vi "自动填充.vi"(5 "填充方式":i32(ring)=1 items=["xlFillCopy"=1, "xlFillDays"=5, "xlFillDefault"=0, "xlFillFormats"=3, "xlFillMonths"=7, "xlFillSeries"=2, "xlFillValues"=4, "xlFillWeekdays"=6, "xlFillYears"=8, "xlGrowthTrend"=10, "xlLinearTrend"=9, "xlFlashFill"=11], 7 "工作表名称":string="Sheet1", 8 "错误输入（无错误）":errorcluster, 11 "单元格区域":T1={"起始列"="A", "起始行"=1, "大小"=[]} {"大小" min=1 max=1048576; "起始行" min=1 max=1048576}) -> (0 "错误输出":errorcluster)   [LabVIEW 2020, in "OperateExcel.lvlib"]
uses:
  OperateExcel.lvlib
  Globals.vi
  <vilib>/Utility/error.llb/Error Cluster From Error Code.vi
  <vilib>/ErrorRing/Error Ring.xnode
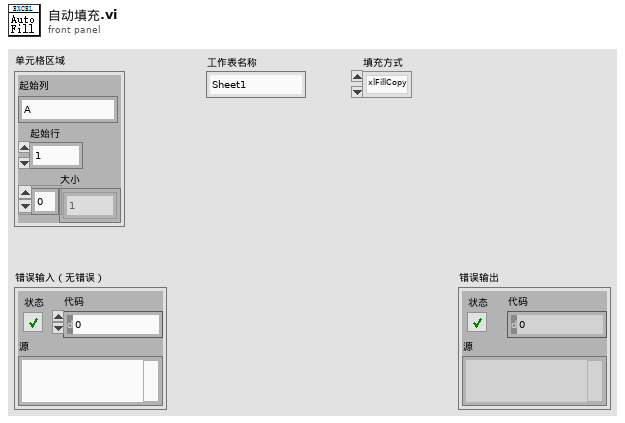
[diagram p1: front panel]
types:
  T1 = typedef "OperateExcel.lvlib/单元格区域.ctl" = cluster{"起始列":string, "起始行":u32, "大小":u32[]}
  T2 = typedef "OperateExcel.lvlib/引用簇.ctl" = cluster{"Excel._Application":refnum<k7>, "Workbooks":refnum<k7>, "Open":refnum<k7>, "Worksheets":refnum<k7>, "sheetList":refnum<k7>[]}
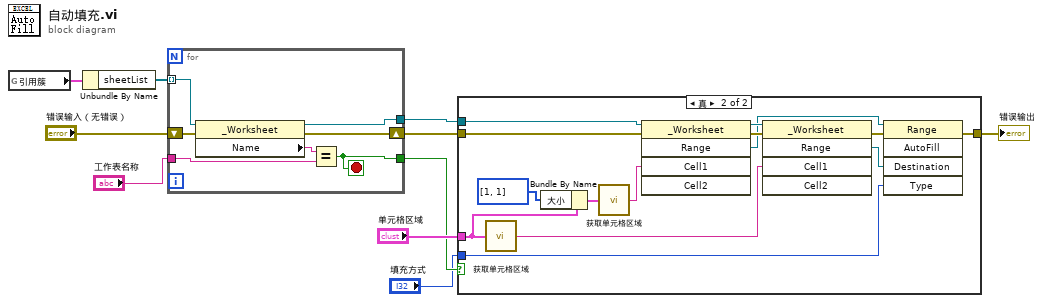
[diagram p0: block diagram]
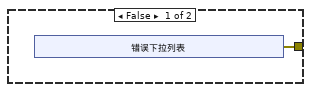
[diagram p2: hidden frame]
diagram:
  n1 = global read "Globals.vi" "引用簇"() -> (w3:T2)
  n2 = Unbundle By Name(w3) -> ("sheetList"=w10:refnum<k7>[])
  n3 = for {
    tunnel: w10 -> [w17] mode=indexing
    tunnel: "工作表名称" -> [w15]
    tunnel: [w14] -> w9
    shift-right: [w12] -> w7
    shift-left: "错误输入（无错误）" -> [w13]
    tunnel: [w11] -> w2
    stop <- w11 stop-if-true
    n4 = property class="_Worksheet"(reference=w17, error in=w13) -> (reference out=w14:refnum<k7>, error out=w12:errorcluster, "Name"=w16:string)
    n5 = Equal?(x=w16, y=w15) -> (x = y?=w11:bool)
  }
  n6 = case shown="真" w2 {
    tunnel: w9 -> [_ w32]
    tunnel: w7 -> [_ w26]
    tunnel: [w18 w35] -> w6
    tunnel: "单元格区域" -> [_ w30]
    tunnel: "填充方式" -> [_ w33]
    frame False {
      n7 = xnode "错误下拉列表"() -> ("错误输出"=w18:errorcluster)
    }
    frame True {
      n8 = call "获取单元格区域.vi"("单元格区域"=w30) -> ("单元格区域"=w34:string)
      n9 = Bundle By Name(cluster=w30, "大小"=u32[] [1, 1]) -> (w29:T1)
      n10 = call "获取单元格区域.vi"("单元格区域"=w29) -> ("单元格区域"=w27:string)
      n11 = invoke class="_Worksheet" method="Range"(reference=w32, error in=w26, "Cell1"=w27) -> (reference out=w31:refnum<k7>, error out=w25:errorcluster, "Range"=w24:refnum<k7>)  [unwired: 2 in, 2 out]
      n12 = invoke class="_Worksheet" method="Range"(reference=w31, error in=w25, "Cell1"=w34) -> (error out=w36:errorcluster, "Range"=w23:refnum<k7>)  [unwired: 2 in, 3 out]
      n13 = invoke on="调用节点" class="Range" method="AutoFill"(reference=w24, error in=w36, "Destination"=w23, "Type"=w33) -> (error out=w35:errorcluster)  [unwired: 1 in, 4 out]
    }
  }
  "错误输出" <- w6
